vi "Parse.vi"(8 "error in (no error)":errorcluster, 10 "Data String":string, 11 "Time Parser in":refnum<class "Time Parser.lvclass">) -> (0 "error out":errorcluster, 2 "Data Values":dbl[](array[numeric]), 3 "Time Parser out":refnum<class "Time Parser.lvclass">)   [LabVIEW 2024, in "Time Parser.lvclass"]
doc: "Time Parserl.lvclass:Parse.vi\n\nThis VI returns a number of possible channels from the Clock Time Bus string.\n\nInstrument Communication Module Version 1.0\nSeptember, 2017 Original Code Consulting David Thomson\n www.originalcode.com"
uses:
  Time Parser.lvclass
  <vilib>/Utility/miscctls.llb/LVDateTimeRec.ctl
  Time Parser.lvclass/Time Parser.ctl
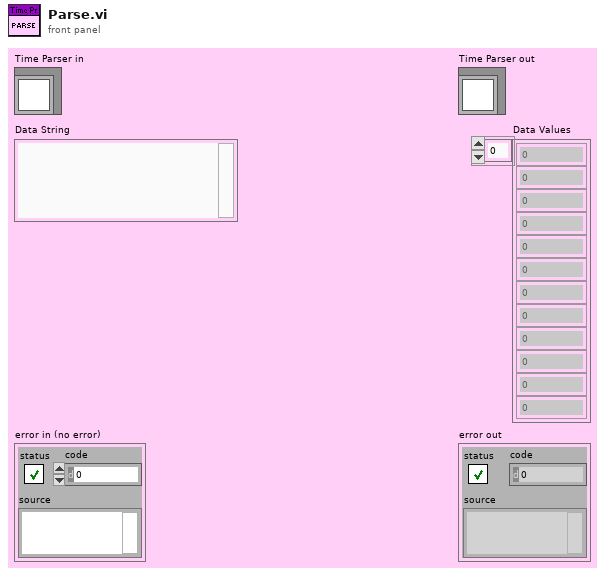
[diagram p1: front panel]
types:
  T1 = typedef "LVDateTimeRec.ctl" = cluster{"fractional second":dbl, "second":i32, "minute":i32, "hour":i32, "day of month":i32, "month":i32, "year":i32, "day of week":i32, "day of year":i32, "DST":i32}
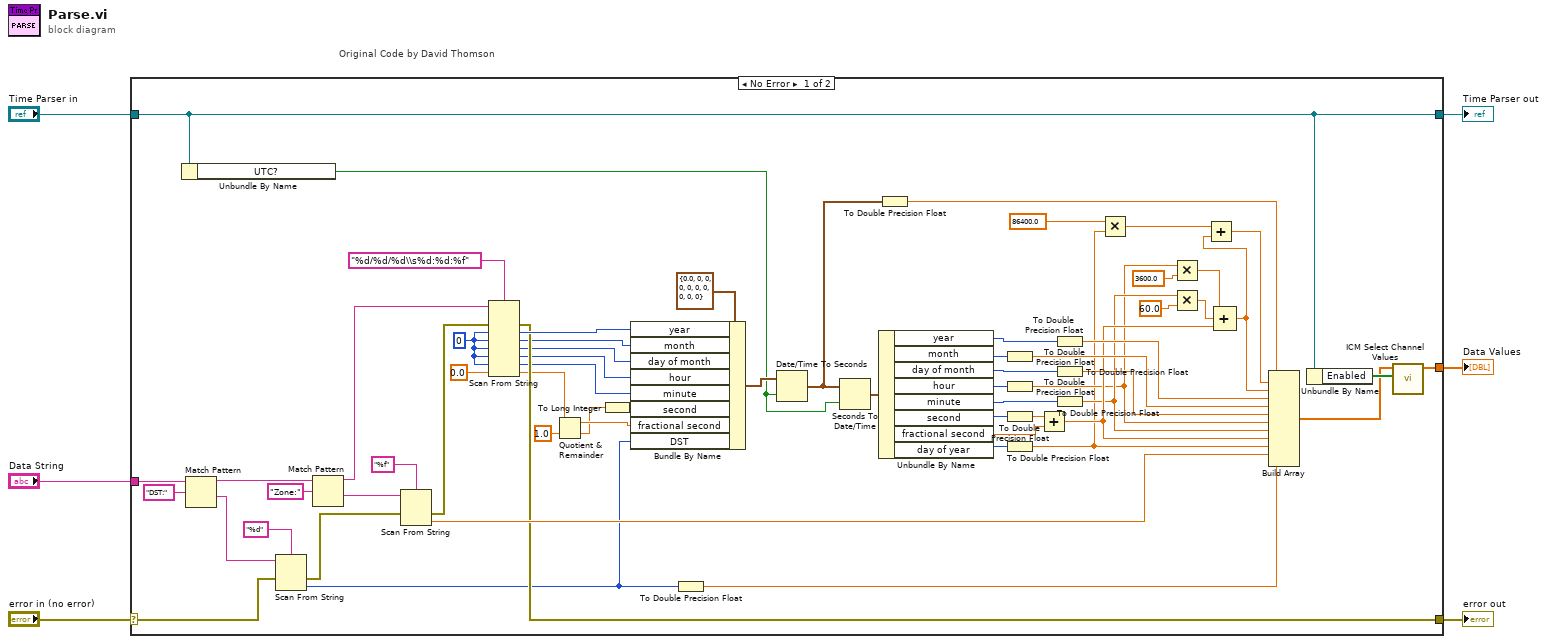
[diagram p0: block diagram]
diagram:
  n1 = case "Original Code by David Thomson" shown="No Error" "error in (no error)" {
    selector: "error in (no error)" -> [w45 w71]
    tunnel: [w44 w71] -> w5
    tunnel: [w17 w70] -> w3
    tunnel: "Time Parser in" -> [w17 w70]
    tunnel: "Data String" -> [w67 _]
    tunnel: [w69 _] -> w1
    frame No Error {
      w59 = 0
      n2 = Unbundle By Name(w17) -> ("UTC?"=w7:bool)
      n3 = Match Pattern(string=w67, regular expression="DST:") -> (before substring=w65:string, after substring=w60:string)  [unwired: 1 in, 2 out]
      n4 = Scan From String(format string="%d", input string=w60, error in=w45) -> (error out=w54:errorcluster, output 1=w8:i32)  [unwired: 2 in, 2 out]
      n5 = Match Pattern(string=w65, regular expression="Zone:") -> (before substring=w55:string, after substring=w61:string)  [unwired: 1 in, 2 out]
      n6 = Scan From String(format string="%f", input string=w61, error in=w54) -> (error out=w53:errorcluster, output 1=w56:dbl)  [unwired: 2 in, 2 out]
      n7 = Scan From String(format string="%d/%d/%d\\s%d:%d:%f", input string=w55, error in=w53, default 1=w59, default 2=w59, default 3=w59, default 4=w59, default 5=w59, default 6=0.0) -> (error out=w44:errorcluster, output 1=w47:i32, output 2=w43:i32, output 3=w42:i32, output 4=w41:i32, output 5=w40:i32, output 6=w39:dbl)  [unwired: 1 in, 2 out]
      n8 = Quotient & Remainder(x=w39, y=1.0) -> (x-y*floor(x/y)=w37:dbl, floor(x/y)=w36:dbl)
      n9 = To Long Integer(number=w36) -> (32bit integer=w35:i32)
      n10 = Bundle By Name(cluster=T1 {"fractional second"=0.0, "second"=0, "minute"=0, "hour"=0, "day of month"=0, "month"=0, "year"=0, "day of week"=0, "day of year"=0, "DST"=0} ("date time rec"), "year"=w47, "month"=w43, "day of month"=w42, "hour"=w41, "minute"=w40, "second"=w35, "fractional second"=w37, "DST"=w8) -> (w49:T1)
      n11 = To Double Precision Float(number=w8) -> (double precision float=w58:dbl)
      n12 = Date/Time To Seconds(1:w7, 2:w49) -> (0:w16:timestamp)
      n13 = Seconds To Date/Time(time stamp (now)=w16, to UTC (F)=w7) -> (date time rec=w50:T1)
      n14 = Unbundle By Name(w50) -> ("year"=w27:i32, "month"=w28:i32, "day of month"=w29:i32, "hour"=w30:i32, "minute"=w31:i32, "second"=w33:i32, "fractional second"=w32:dbl, "day of year"=w51:i32)
      n15 = To Double Precision Float(number=w16) -> (double precision float=w15:dbl)
      n16 = To Double Precision Float(number=w28) -> (double precision float=w25:dbl)
      n17 = To Double Precision Float(number=w30) -> (double precision float=w18:dbl)
      n18 = To Double Precision Float(number=w33) -> (double precision float=w34:dbl)
      n19 = To Double Precision Float(number=w51) -> (double precision float=w13:dbl)
      n20 = Add(x=w34, y=w32) -> (x+y=w20:dbl)
      n21 = To Double Precision Float(number=w27) -> (double precision float=w24:dbl)
      n22 = To Double Precision Float(number=w29) -> (double precision float=w26:dbl)
      n23 = To Double Precision Float(number=w31) -> (double precision float=w19:dbl)
      n24 = Multiply(x=86400.0 ("y"), y=w13) -> (x*y=w11:dbl)
      n25 = Multiply(x=w18, y=3600.0) -> (x*y=w14:dbl)
      n26 = Multiply(x=w19, y=60.0) -> (x*y=w21:dbl)
      n27 = Compound Arithmetic op=ADD(w14, w21, w20) -> (w9:dbl)
      n28 = Add(x=w11, y=w9) -> (x+y=w10:dbl)
      n29 = Build Array(w15, w10, w9, w24, w25, w26, w18, w19, w20, w13, w56, w58) -> (w57:dbl[])
      n30 = Unbundle By Name(w17) -> ("Enabled"=w68:bool[])
      n31 = call "ICM Select Channel Values.vi"("Enabled"=w68, "Channel Values"=w57) -> ("Enabled Values"=w69:dbl[])  [unwired: 9 in]
    }
    frame Error {
    }
  }
  "error out" <- w5
  "Time Parser out" <- w3
  "Data Values" <- w1
